vi "Load All Values and Start SCHMPS2 FPGA.vi"(8 "error in":errorcluster) -> (0 "error out":errorcluster, 2 "Data Size":i32, 3 "Refnum out":T1)   [LabVIEW 2020]
doc: "Author: Scott Hannahs <sth@magnet.fsu.edu>\nCopyright 2018 Florida State University, All rights reserved."
uses:
  <vilib>/rvi/interface/nirviReadWriteControl/nirviReadWriteControl.xnode
  <vilib>/rvi/interface/nirviMethod/nirviMethod.xnode
  <vilib>/FPGAPlugInAG/Dynamic/niLvFpga_Run_Dynamic.vi
  <vilib>/rvi/interface/Simulation/niFpgaSimulationCallBeginRW.vi
  <vilib>/rvi/errors/niLvFpgaAdjustHostInterfaceError.vi
  <vilib>/rvi/interface/nirviOpenFPGA/nirviOpenFPGA.xnode
  <vilib>/FPGAPlugInAG/Dynamic/niLvFpga_ConfigureFifo_Dynamic.vi
  <vilib>/rvi/errors/niLvFpgaMergeErrorWithErrorCode.vi
  <vilib>/FPGAPlugInAG/Dynamic/niLvFpga_StartFifo_Dynamic.vi
  NiFpgaLv.dll
  RT Controls/FPGA SCH Secondary Digitizer Ref.ctl
  FPGA Bitfiles/SCHProtection_SCHMPSSecondaryF_SecondaryFPGADig_T6ps523+tyQ.lvbitx
  <vilib>/FPGAPlugInAG/cRIO-9039/niLvFpga_Open_cRIO-9039.vi
  <vilib>/rvi/interface/common/dynamic/niFpgaDynamicAddResources.vi
panel:
  out "Build":u8=57
  out "Fix":u8=2
  out "Minor":u8=2
  out "Major":u8=2
  out "Actual Depth":u32
  # "."
  # "."
  # "."
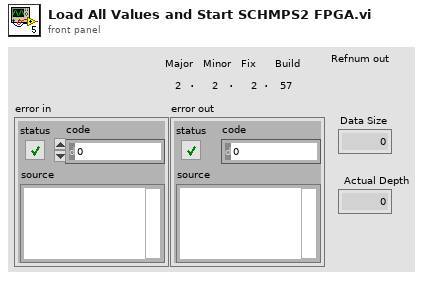
[diagram p1: front panel]
types:
  T1 = typedef "FPGA SCH Secondary Digitizer Ref.ctl" = refnum<k20>
  T2 = enum16{"Input Voltage", "Zero Voltage", "Calibrate Voltage"}
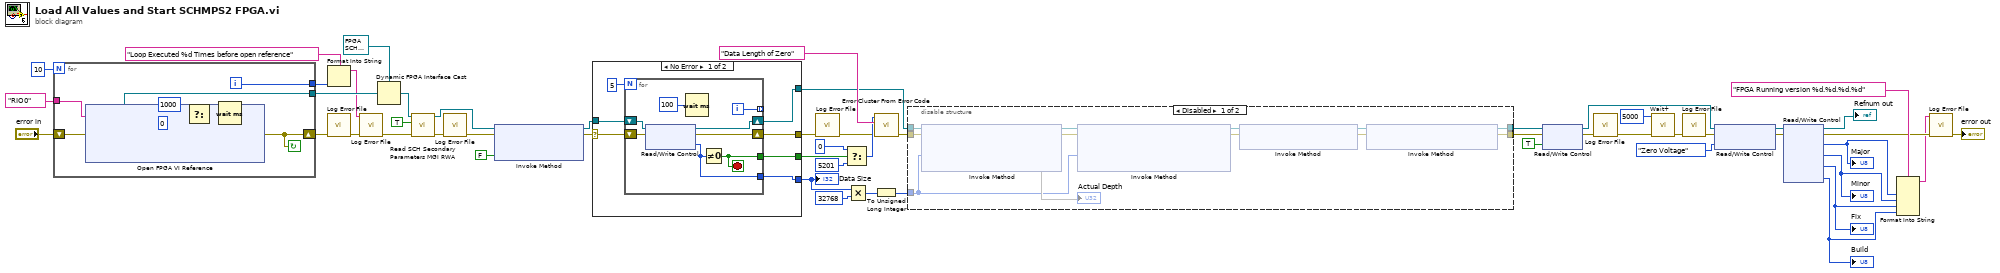
[diagram p0: block diagram]
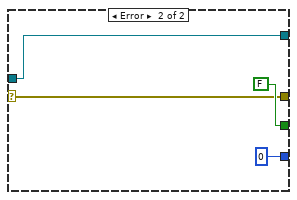
[diagram p3: hidden frame]
diagram:
  n1 = for {
    N: 10 -> [_]
    tunnel: [w60] -> w38
    tunnel: tag "RIO0" ("resource name") -> [w59]
    shift-right: [w54] -> w30
    shift-left: "error in" -> [w61]
    tunnel: [w55] -> w20
    i -> [w55]
    stop <- w54 continue-if-true
    n2 = xnode "Open FPGA VI Reference"("error in"=w61, "resource name"=w59) -> ("FPGA VI Reference Out"=w60:refnum<k20>, "error out"=w54:errorcluster)
    n3 = Select(t=u32 1000, s=w54, f=u32 0 ("milliseconds to wait")) -> (s? t:f=w58:u32)
    n4 = Wait (ms)(milliseconds to wait=w58) -> ()  [unwired: 1 out]
  }
  n5 = Format Into String(format string="Loop Executed %d Times before open reference", w20) -> (resulting string=w16:string)  [unwired: 2 in, 1 out]
  n6 = call "Log Error File.vi"("error in (no error)"=w30) -> ("error out"=w18:errorcluster)  [unwired: 10 in]
  n7 = call "Log Error File.vi"("error in (no error)"=w18, "Log String"=w16) -> ("error out"=w17:errorcluster)  [unwired: 9 in]
  n8 = Dynamic FPGA Interface Cast(Session In=T1 refnum ("Refnum out"), Type=w38) -> (Session Out=w2:T1)
  n9 = call "Read SCH Secondary Parameters MGI RWA.vi"("error in (no error)"=w17, "Done"=TRUE, "FPGA Refnum in"=w2) -> ("error out"=w15:errorcluster, "Refnum out"=w34:T1)  [unwired: 7 in]
  n10 = call "Log Error File.vi"("error in (no error)"=w15) -> ("error out"=w14:errorcluster)  [unwired: 10 in]
  n11 = xnode "Invoke Method"("FPGA VI Reference In"=w34, "error in"=w14, "Wait Until Done (F)"=FALSE) -> ("FPGA VI Reference Out"=w37:T1, "error out"=w45:errorcluster)
  n12 = case shown="No Error" w45 {
    selector: w45 -> [w62 w77]
    tunnel: [w67 w77] -> w13
    tunnel: [w66 FALSE] -> w50
    tunnel: w37 -> [w65 w80]
    tunnel: [w64 w80] -> w36
    tunnel: [w63 0 ("Data Size")] -> w39
    frame No Error {
      n13 = for {
        N: 5 -> [_]
        tunnel: [w70] -> w63
        shift-right: [w71] -> w67
        shift-left: w62 -> [w72]
        shift-right: [w73] -> w64
        shift-left: w65 -> [w74]
        tunnel: [w75] -> w66
        tunnel: [w69] -> _ mode=indexing
        i -> [w69]
        stop <- w75 stop-if-true
        n14 = xnode "Read/Write Control"("FPGA VI Reference In"=w74, "error in"=w72) -> ("FPGA VI Reference Out"=w73:T1, "error out"=w71:errorcluster, "Data Size"=w70:i32)
        n15 = Wait (ms)(milliseconds to wait=u32 100) -> ()  [unwired: 1 out]
        n16 = Not Equal To 0?(x=w70) -> (x != 0?=w75:bool)
      }
    }
    frame Error {
    }
  }
  "Data Size" <- w39
  n17 = call "Log Error File.vi"("error in (no error)"=w13) -> ("error out"=w12:errorcluster)  [unwired: 10 in]
  n18 = Select(t=0, s=w50, f=5201) -> (s? t:f=w48:i32)
  n19 = Multiply(x=w39, y=32768) -> (x*y=w43:i32)
  n20 = To Unsigned Long Integer(number=w43) -> (unsigned 32bit integer=w42:u32)
  n21 = call <vilib>:"Error Cluster From Error Code.vi"("error in (no error)"=w12, "error message (\"\")"="Data Length of Zero" ("error message (\"\")"), "error code (0)"=w48) -> ("error out"=w40:errorcluster)  [unwired: 6 in]
  n22 = disable-structure shown="Disabled" {
    disable-tunnel: w42 -> [w81 _]
    disable-tunnel: w40 -> [w88 w93]
    disable-tunnel: w36 -> [w87 w94]
    disable-tunnel: [w83 w94] -> w35
    disable-tunnel: [w82 w93] -> w32
    frame Disabled {
      n23 = xnode "Invoke Method"("FPGA VI Reference In"=w87, "error in"=w88, "Requested Depth"=w81) -> ("FPGA VI Reference Out"=w86:T1, "error out"=w91:errorcluster, "Actual Depth"=→"Actual Depth")
      n24 = xnode "Invoke Method"("FPGA VI Reference In"=w86, "error in"=w91, "Requested Depth"=w81) -> ("FPGA VI Reference Out"=w85:T1, "error out"=w90:errorcluster)  [unwired: 1 out]
      n25 = xnode "Invoke Method"("FPGA VI Reference In"=w85, "error in"=w90) -> ("FPGA VI Reference Out"=w84:T1, "error out"=w89:errorcluster)
      n26 = xnode "Invoke Method"("FPGA VI Reference In"=w84, "error in"=w89) -> ("FPGA VI Reference Out"=w83:T1, "error out"=w82:errorcluster)
    }
    frame Enabled {
    }
  }
  n27 = xnode "Read/Write Control"("FPGA VI Reference In"=w35, "error in"=w32, "Reset"=TRUE) -> ("FPGA VI Reference Out"=w6:T1, "error out"=w7:errorcluster)
  n28 = call "Log Error File.vi"("error in (no error)"=w7) -> ("error out"=w4:errorcluster)  [unwired: 10 in]
  n29 = call "Wait+.vi"("Error In"=w4, "milliseconds to wait"=u32 5000) -> ("Error Out"=w3:errorcluster)  [unwired: 4 in, 1 out]
  n30 = call "Log Error File.vi"("error in (no error)"=w3) -> ("error out"=w11:errorcluster)  [unwired: 10 in]
  n31 = xnode "Read/Write Control"("FPGA VI Reference In"=w6, "error in"=w11, "Input Select"=T2."Zero Voltage") -> ("FPGA VI Reference Out"=w31:T1, "error out"=w26:errorcluster)
  n32 = xnode "Read/Write Control"("FPGA VI Reference In"=w31, "error in"=w26) -> ("FPGA VI Reference Out"=→"Refnum out":T1, "error out"=w9:errorcluster, "Major"=w25:u8, "Minor"=w24:u8, "Fix"=w23:u8, "Build"=w22:u8)
  "Major" <- w25
  "Minor" <- w24
  "Fix" <- w23
  "Build" <- w22
  n33 = Format Into String(format string="FPGA Running version %d.%d.%d.%d", w25, w24, w23, w22) -> (resulting string=w8:string)  [unwired: 2 in, 1 out]
  n34 = call "Log Error File.vi"("error in (no error)"=w9, "Log String"=w8) -> ("error out"=→"error out":errorcluster)  [unwired: 9 in]
